vi "DUT Main.vi"(11 "DUT HW Resources":T3={"CAN Interface"="CAN2", "CAN Termination"=TRUE, "Digital Counter"="PXI1Slot8/ctr0", "DO Terminals"=["/PXI1Slot8/PFI0", "/PXI1Slot8/PFI1", "/PXI1Slot8/PFI2", "/PXI1Slot8/PFI3", "/PXI1Slot8/PFI4", "/PXI1Slot8/PFI5", "/PXI1Slot8/PFI6", "/PXI1Slot8/PFI7"]}) -> ()   [LabVIEW 2023]
uses:
  DUT Sample/DUT Sample.lvclass
  DUT Sample/typedefs/DO Finite Pulse Config.ctl
  DUT Sample/typedefs/DUT HW Resources.ctl
  DUT Sample/typedefs/DUT Command Type.ctl
  DUT Sample/typedefs/DUT Command.ctl
panel:
  out "init error":errorcluster
  out "error command":errorcluster
  out "Processing Commands":T1[](array[typedef])
  out "error out":errorcluster
  in  "Stop":bool
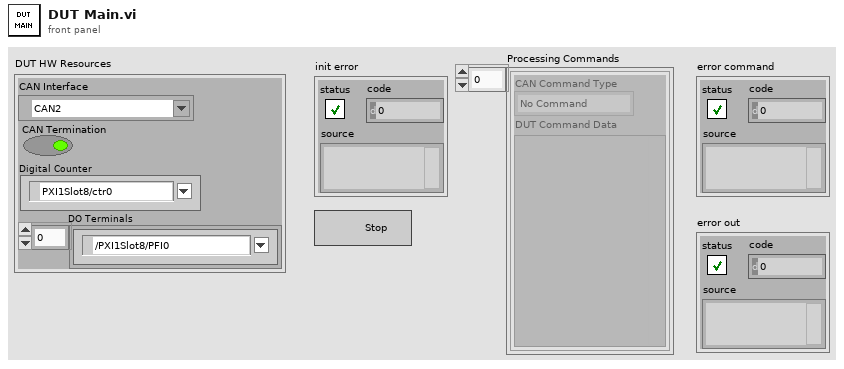
[diagram p1: front panel]
types:
  T1 = typedef "DUT Sample.lvclass/DUT Command.ctl" = cluster{"CAN Command Type":T2, "DUT Command Data":variant}
  T2 = typedef "DUT Sample.lvclass/DUT Command Type.ctl" = enum16{"No Command", "Generate DO Pulse"}
  T3 = typedef "DUT Sample.lvclass/DUT HW Resources.ctl" = cluster{"CAN Interface":refnum<k21>, "CAN Termination":bool, "Digital Counter":tag, "DO Terminals":tag[]}
  T4 = typedef "DUT Sample.lvclass/DO Finite Pulse Config.ctl" = cluster{"Port Number":u8, "Number of Pulses":u8, "High Time (ms)":u16, "Low Time (ms)":u16}
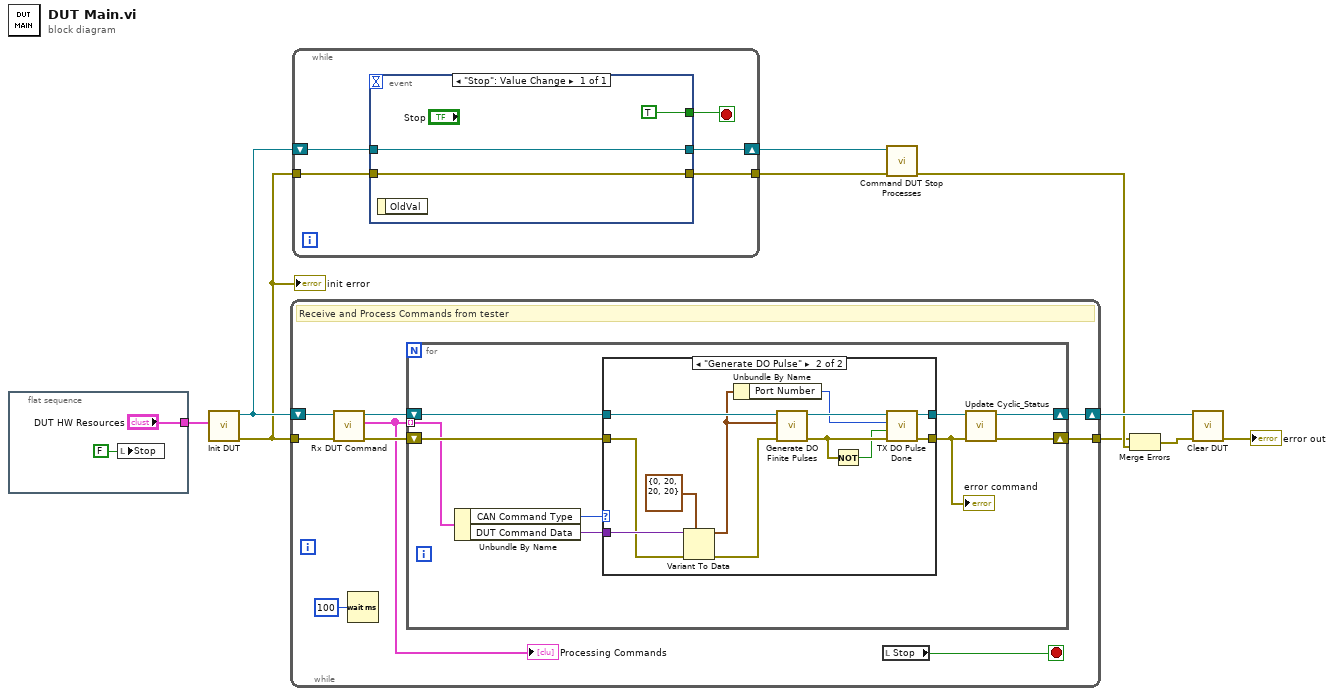
[diagram p0: block diagram]
diagram:
  n1 = flat-sequence {
    tunnel: ["DUT HW Resources"] -> w8
    frame #0 {
      n2 = local write "Stop"(FALSE ("Stop")) -> ()
    }
  }
  n3 = call "Init DUT.vi"("DUT HW Resources"=w8) -> ("error out"=w1:errorcluster, "DUT Sample out"=w7:refnum<class "DUT Sample.lvclass">)  [unwired: 9 in]
  "init error" <- w1
  n4 = while {
    shift-right: [w17] -> w10
    shift-left: w7 -> [w21]
    tunnel: w1 -> [w20]
    tunnel: [w16] -> w2
    stop <- w15 stop-if-true
    # "Receive and Process Commands from tester"
    n5 = call "Rx DUT Command.vi"("error in (no error)"=w20, "DUT Sample in"=w21) -> ("error out"=w18:errorcluster, "Commands"=w13:T1[], "DUT Sample out"=w19:refnum<class "DUT Sample.lvclass">)  [unwired: 7 in]
    "Processing Commands" <- w13
    n6 = Wait (ms)(milliseconds to wait=u32 100) -> ()  [unwired: 1 out]
    n7 = for {
      shift-right: [w23] -> w17
      shift-left: w19 -> [w29]
      shift-right: [w25] -> w16
      shift-left: w18 -> [w28]
      tunnel: w13 -> [w26] mode=indexing
      n8 = Unbundle By Name(w26) -> ("CAN Command Type"=w30:T2, "DUT Command Data"=w27:variant)
      n9 = case shown="\"Generate DO Pulse\"" w30 {
        tunnel: [w32 w37] -> w24
        tunnel: w29 -> [w32 w44]
        tunnel: w28 -> [w31 w42]
        tunnel: [w31 w39] -> w22
        tunnel: w27 -> [_ w43]
        frame "No Command", Default {
        }
        frame "Generate DO Pulse" {
          n10 = Variant To Data(error in=w42, type=T4 {"Port Number"=0, "Number of Pulses"=20, "High Time (ms)"=20, "Low Time (ms)"=20} ("DO Finite Pulse Config"), Variant=w43) -> (data=w36:T4, error out=w40:errorcluster)
          n11 = Unbundle By Name(w36) -> ("Port Number"=w35:u8)
          n12 = call "Generate DO Finite Pulses.vi"("error in"=w40, "DO Finite Pulse Config"=w36, "DUT Sample in"=w44) -> ("error out"=w34:errorcluster, "DUT Sample out"=w38:refnum<class "DUT Sample.lvclass">)  [unwired: 7 in]
          n13 = Not(x=w34) -> (.not. x?=w33:bool)
          n14 = call "TX DO Pulse Done.vi"("error in (no error)"=w34, "Success?"=w33, "Port Number"=w35, "DUT Sample in"=w38) -> ("error out"=w39:errorcluster, "DUT Sample out"=w37:refnum<class "DUT Sample.lvclass">)  [unwired: 6 in]
        }
      }
      "error command" <- w22
      n15 = call "Update Cyclic_Status.vi"("error in (no error)"=w22, "DUT Sample in"=w24) -> ("error out"=w25:errorcluster, "DUT Sample out"=w23:refnum<class "DUT Sample.lvclass">)  [unwired: 8 in]
    }
    n16 = local read "Stop"() -> (w15:bool)
  }
  n17 = while {
    tunnel: w1 -> [w47]
    tunnel: [w46] -> w5
    shift-right: [w45] -> w3
    shift-left: w7 -> [w48]
    stop <- w49 stop-if-true
    n18 = event shown="[0] \"Stop\": Value Change" {
      selector: _ -> [_]
      dyn-events: _ -> [_]
      timeout: _ -> [_]
      tunnel: [TRUE] -> w49
      tunnel: w48 -> [w50]
      tunnel: w47 -> [w51]
      tunnel: [w51] -> w46
      tunnel: [w50] -> w45
      event "Stop": Value Change {
        n19 = event-data() -> ()  [unwired: 1 in, 1 out]
      }
    }
  }
  n20 = call "Command DUT Stop Processes.vi"("error in (no error)"=w5, "DUT Sample in"=w3) -> ("error out"=w4:errorcluster)  [unwired: 8 in, 1 out]
  n21 = Merge Errors(w2, w4) -> (w6:errorcluster)
  n22 = call "Clear DUT.vi"("error in (no error)"=w6, "DUT Sample in"=w10) -> ("error out"=→"error out":errorcluster)  [unwired: 9 in]
